vi "Modelo3d.vi"(9 "String 2":string, 10 "String":string, 11 "SceneGraphDisplay in":refnum<vi>) -> (3 "SceneNode out":refnum<vi>(3d-picture))   [LabVIEW 2023]
uses:
  <vilib>/Utility/miscctls.llb/LV3DPointTypeDef.ctl
  <vilib>/picture/3D Picture Control/Object/Add Object (no reference).vi
  <vilib>/picture/3D Picture Control/Object/Create Object (name).vi
  <vilib>/picture/3D Picture Control/NI_3D Picture Control.lvlib
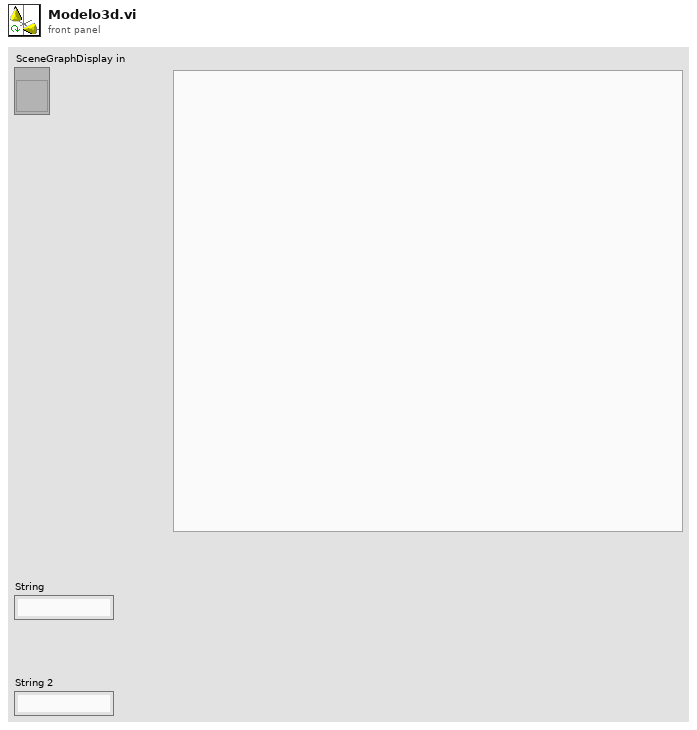
[diagram p1: front panel]
types:
  T1 = typedef "LV3DPointTypeDef.ctl" = cluster{"X":sgl, "Y":sgl, "Z":sgl}
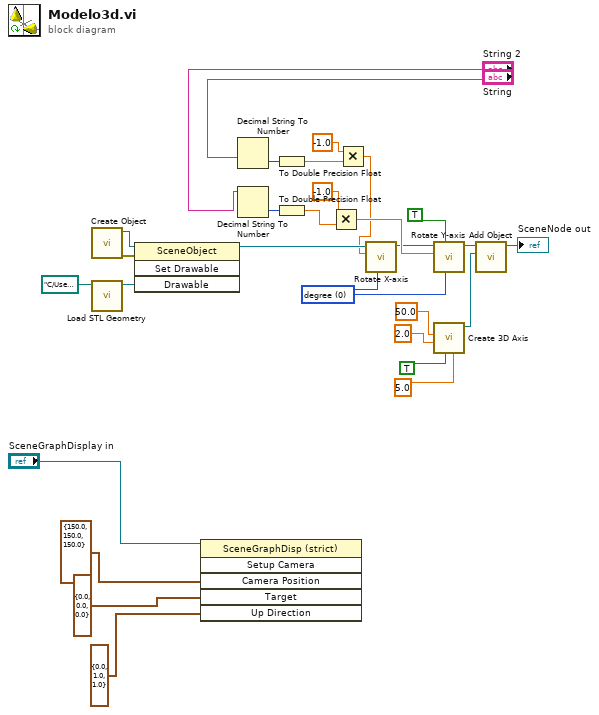
[diagram p0: block diagram]
diagram:
  w15 = u16 0 items=["degree", "radians"] ("angle unit")
  n1 = call-poly <vilib>:"Create Object.vi"() -> ("error out"=w4:errorcluster, "Scene:New Object"=w3:refnum<vi>)  [unwired: 10 in]
  n2 = call <vilib>:"Load STL Geometry.vi"("Model File"=path "C:/Users/SNGULAR/Downloads/Powerful Snaget.stl") -> ("New Mesh Refnum"=w11:refnum<vi>)  [unwired: 9 in, 1 out]
  n3 = invoke class="SceneObject" method="Set Drawable"(reference=w3, error in=w4, "Drawable"=w11) -> (reference out=w29:refnum<vi>)  [unwired: 1 in, 3 out]
  n4 = invoke on="Invoke Node" class="SceneGraphDisp (strict)" method="Setup Camera"(reference="SceneGraphDisplay in", "Camera Position"=T1 {"X"=150.0, "Y"=150.0, "Z"=150.0}, "Target"=T1 {"X"=0.0, "Y"=0.0, "Z"=0.0}, "Up Direction"=T1 {"X"=0.0, "Y"=1.0, "Z"=1.0}) -> ()  [unwired: 2 in, 6 out]
  n5 = Decimal String To Number(string="String") -> (number=w16:i32)  [unwired: 2 in, 1 out]
  n6 = Decimal String To Number(string="String 2") -> (number=w2:i32)  [unwired: 2 in, 1 out]
  n7 = To Double Precision Float(number=w16) -> (double precision float=w19:dbl)
  n8 = To Double Precision Float(number=w2) -> (double precision float=w23:dbl)
  n9 = Multiply(x=-1.0, y=w23) -> (x*y=w24:dbl)
  n10 = Multiply(x=-1.0, y=w19) -> (x*y=w20:dbl)
  n11 = call <vilib>:"Rotate X-axis.vi"("angle unit"=w15, "angle"=w20, "Scene Object In"=w29) -> ("Scene Object Out"=w9:refnum<vi>)  [unwired: 7 in, 1 out]
  n12 = call <vilib>:"Rotate Y-axis.vi"("angle unit"=w15, "Relative?"=TRUE, "angle"=w24, "Scene Object In"=w9) -> ("Scene Object Out"=w27:refnum<vi>)  [unwired: 6 in, 1 out]
  n13 = call <vilib>:"Create 3D Axis.vi"("Character Size"=sgl 5.0, "Axis label?"=TRUE, "Radius"=sgl 2.0, "Length"=sgl 50.0) -> ("New Object Refnum"=w18:refnum<vi>)  [unwired: 6 in, 1 out]
  n14 = call-poly <vilib>:"Add Object.vi"("New Object In"=w18, "Scene Object In"=w27) -> ("Scene Object Out"=→"SceneNode out":refnum<vi>)  [unwired: 8 in, 1 out]
